vi "Read pAvailable.vi"(8 "error in (no error)":errorcluster, 11 "bbPlayers in":refnum<class "bbPlayers.lvclass">) -> (0 "error out":errorcluster, 2 "pAvailable":bool, 3 "bbPlayers out":refnum<class "bbPlayers.lvclass">)   [LabVIEW 2020, in "bbPlayers.lvclass"]
doc: "Read the current value of pAvailable."
uses:
  bbPlayers.lvclass
  bbPlayers.lvclass/bbPlayers.ctl
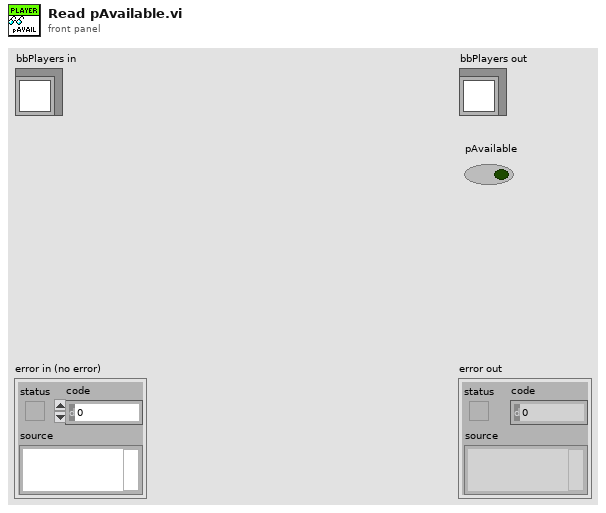
[diagram p1: front panel]
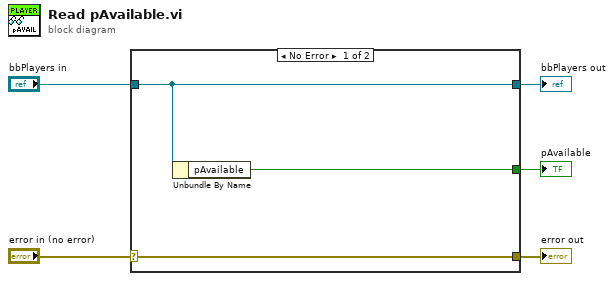
[diagram p0: block diagram]
diagram:
  n1 = case shown="No Error" "error in (no error)" {
    selector: "error in (no error)" -> [w8 w9]
    tunnel: [w8 w9] -> w4
    tunnel: [w7 w10] -> w2
    tunnel: "bbPlayers in" -> [w7 w10]
    tunnel: [w6 _] -> w1
    frame No Error {
      n2 = Unbundle By Name(w7) -> ("pAvailable"=w6:bool)
    }
    frame Error {
    }
  }
  "error out" <- w4
  "bbPlayers out" <- w2
  "pAvailable" <- w1
